vi "Flatten.vi"(8 "error in":errorcluster, 9 "Data":T1) -> (0 "error out":errorcluster, 2 "Buffer":u8[](array[numeric]) format="%.0x")   [LabVIEW 2020, in "StartLog.lvlib"]
uses:
  StartLog.lvlib
  Data.ctl
  lv-protoc/LV-Proto/LV-Proto.lvlib
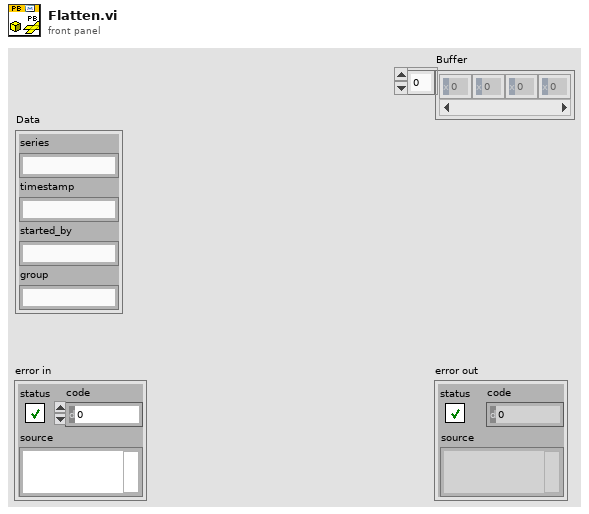
[diagram p1: front panel]
types:
  T1 = typedef "StartLog.lvlib/Data.ctl" = cluster{"series":string, "timestamp":string, "started_by":string, "group":string}
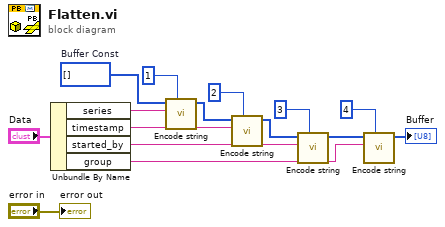
[diagram p0: block diagram]
diagram:
  w13 = u8[] []  # Buffer Const
  n1 = Unbundle By Name("Data") -> ("series"=w11:string, "timestamp"=w8:string, "started_by"=w5:string, "group"=w2:string)
  n2 = call "Encode string.vi"("Field Number"=1, "string"=w11, "Buffer in"=w13) -> ("Buffer"=w10:u8[])  [unwired: 8 in]
  n3 = call "Encode string.vi"("Field Number"=2, "string"=w8, "Buffer in"=w10) -> ("Buffer"=w7:u8[])  [unwired: 8 in]
  n4 = call "Encode string.vi"("Field Number"=3, "string"=w5, "Buffer in"=w7) -> ("Buffer"=w4:u8[])  [unwired: 8 in]
  n5 = call "Encode string.vi"("Field Number"=4, "string"=w2, "Buffer in"=w4) -> ("Buffer"=→"Buffer":u8[])  [unwired: 8 in]
  "error out" <- "error in"
